vi "Initialize Attributes.vi"(8 "error in (no error)":errorcluster, 10 "Attribute Data":variant, 11 "CS++PVProxy in":refnum<class "CS++PVProxy.lvclass">) -> (0 "error out":errorcluster, 2 "Found?":bool, 3 "CS++PVProxy out":refnum<class "CS++PVProxy.lvclass">)   [LabVIEW 2015, in "CS++PVProxy.lvlib" / "CS++PVProxy.lvclass"]
doc: "Initialize object attribute.\n\nUnique resources should be allocated elsewhere!"
uses:
  CS++PVProxy.lvclass
  Classes/CS++ProcessVariables/ProcessVariable/PV.lvclass
  CS++PVMonitor Messages/CS++PVUpdate Msg/CS++PVUpdate Msg.lvclass
  CS++BaseActor/CS++BaseActor.lvclass/CS++BaseActor.ctl
  Classes/CS++ProcessVariables/ProcessVariable/PV.lvclass/PV.ctl
  Classes/CS++ProcessVariables/PVConnection/PVConnection.lvclass
  CS++PVMonitor Messages/CS++PVUpdate Msg/CS++PVUpdate Msg.lvclass/CS++PVUpdate Msg.ctl
  CS++PVProxy.lvclass/CS++PVProxy.ctl
  Classes/CS++ProcessVariables/ProcessVariable/Write Name.vi
  Classes/CS++ProcessVariables/ProcessVariable/Write PV URL.vi
  Classes/CS++ProcessVariables/ProcessVariable/Write Type Descriptor.vi
  <vilib>/Utility/error.llb/Error Cluster From Error Code.vi
  CS++BaseActor/CS++BaseActor.lvclass
  Classes/CS++BaseClasses/Factory/CS++Factory.lvclass
  Libraries/Utilities/CS++Utilities.lvlib
  Classes/CS++ProcessVariables/CS++ProcessVariables.lvlib
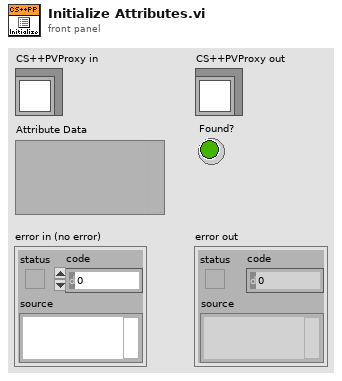
[diagram p1: front panel]
types:
  T1 = cluster{string, string, "CS++PVUpdate Msg out":refnum<class "CS++PVUpdate Msg.lvclass">, "CS++ProcessVariables.lvlib:PVConnection.lvclass":refnum<class "PVConnection.lvclass">}
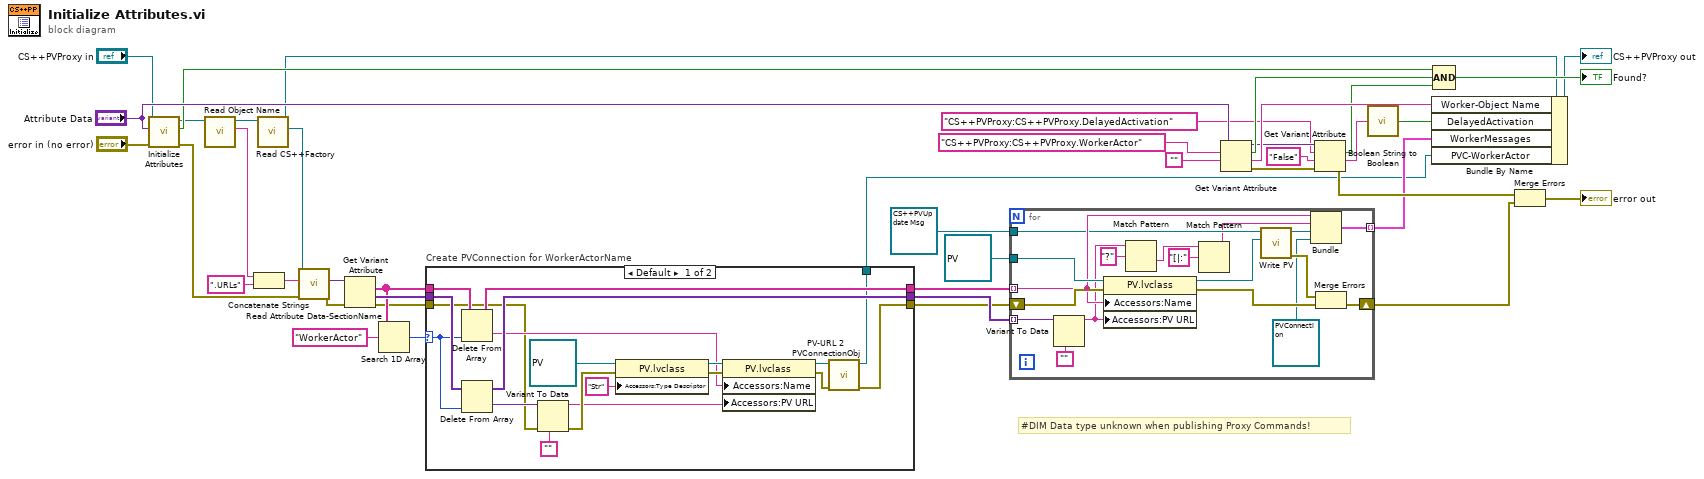
[diagram p0: block diagram]
diagram:
  # "#DIM Data type unknown when publishing Proxy Commands!"
  n1 = call-parent "Initialize Attributes.vi"("error in (no error)"="error in (no error)", "Attribute Data"="Attribute Data", "CS++BaseActor in"="CS++PVProxy in") -> ("error out"=w26:errorcluster, "Found?"=w34:bool, "CS++BaseActor out"=w31:refnum<class "CS++PVProxy.lvclass">)  [unwired: 6 in]
  n2 = call "Read Object Name.vi"("CS++BaseActor in"=w31) -> ("Object Name"=w27:string, "CS++BaseActor out"=w32:refnum<class "CS++PVProxy.lvclass">)  [unwired: 8 in, 1 out]
  n3 = Concatenate Strings(w27, ".URLs" ("string")) -> (w29:string)
  n4 = call "Read CS++Factory.vi"("CS++BaseActor in"=w32) -> ("CS++Factory"=w28:refnum<class "CS++Factory.lvclass">, "CS++BaseActor out"=w20:refnum<class "CS++PVProxy.lvclass">)  [unwired: 8 in, 1 out]
  n5 = call-dynamic "Read Attribute Data-SectionName.vi"("error in (no error)"=w26, "Object Name"=w29, "CS++Factory in"=w28) -> ("error out"=w24:errorcluster, "Attribute Data"=w23:variant)  [unwired: 6 in, 1 out]
  n6 = Get Variant Attribute(Variant=w23, error in=w24) -> (names=w7:string[], values=w9:variant[], error out=w3:errorcluster)  [unwired: 2 in, 1 out]
  n7 = Search 1D Array(1D array=w7, element="WorkerActor") -> (index of element=w5:i32)  [unwired: 1 in]
  n8 = case "Create PVConnection for WorkerActorName" shown="Default" w5 {
    selector: w5 -> [w57 _]
    tunnel: w9 -> [w61 w63]
    tunnel: [w60 w63] -> w8
    tunnel: w7 -> [w59 w64]
    tunnel: [w58 w64] -> w6
    tunnel: w3 -> [w47 w62]
    tunnel: [w45 w62] -> w2
    tunnel: [w44 _] -> w1
    frame Default {
      n9 = Delete From Array(array=w59, index=w57) -> (deleted portion=w48:string, array with subset deleted=w58:string[])  [unwired: 1 in]
      n10 = Delete From Array(array=w61, index=w57) -> (deleted portion=w49:variant, array with subset deleted=w60:variant[])  [unwired: 1 in]
      n11 = Variant To Data(error in=w47, type="", Variant=w49) -> (data=w43:string, error out=w46:errorcluster)
      n12 = property class="PV.lvclass"(reference=refnum<class "PV.lvclass"> refnum ("CS++ProcessVariables.lvlib:PV.lvclass"), error in=w46, "Accessors:Type Descriptor"="Str" ("Type Descriptor")) -> (reference out=w55:refnum<class "PV.lvclass">, error out=w56:errorcluster)
      n13 = property class="PV.lvclass"(reference=w55, error in=w56, "Accessors:Name"=w48, "Accessors:PV URL"=w43) -> (reference out=w53:refnum<class "PV.lvclass">, error out=w54:errorcluster)
      n14 = call "PV-URL 2 PVConnectionObj.vi"("Error In"=w54, "PV"=w53) -> ("Error Out"=w45:errorcluster, "PVConnection"=w44:refnum<class "PVConnection.lvclass">)  [unwired: 7 in, 1 out]
    }
    frame -1 {
    }
  }
  n15 = for {
    tunnel: refnum<class "PV.lvclass"> refnum ("CS++ProcessVariables.lvlib:PV.lvclass") -> [w82]
    shift-right: [w72] -> w22
    shift-left: w2 -> [w79]
    tunnel: w6 -> [w78] mode=indexing
    tunnel: w8 -> [w80] mode=indexing
    tunnel: [w77] -> w11 mode=indexing
    tunnel: refnum<class "CS++PVUpdate Msg.lvclass"> refnum ("CS++PVMonitor.lvlib:CS++PVUpdate Msg.lvclass") -> [w76]
    n16 = Variant To Data(type="", Variant=w80) -> (data=w68:string)  [unwired: 1 in, 1 out]
    n17 = property class="PV.lvclass"(reference=w82, error in=w79, "Accessors:Name"=w78, "Accessors:PV URL"=w68) -> (reference out=w74:refnum<class "PV.lvclass">, error out=w71:errorcluster)
    n18 = Match Pattern(string=w68, regular expression="?") -> (after substring=w65:string)  [unwired: 1 in, 3 out]
    n19 = Match Pattern(string=w65, regular expression="[|:") -> (before substring=w67:string)  [unwired: 1 in, 3 out]
    n20 = call "Write PV.vi"("PV"=w74, "CS++PVUpdate Msg in"=w76) -> ("error out"=w73:errorcluster, "CS++PVUpdate Msg out"=w75:refnum<class "CS++PVUpdate Msg.lvclass">)  [unwired: 8 in]
    n21 = Bundle(w78, w67, "CS++PVUpdate Msg out"=w75, "CS++ProcessVariables.lvlib:PVConnection.lvclass"=refnum<class "PVConnection.lvclass"> refnum) -> (w77:T1)  [unwired: 1 in]
    n22 = Merge Errors(w73, w71) -> (w72:errorcluster)
  }
  n23 = Get Variant Attribute(Variant="Attribute Data", name="CS++PVProxy:CS++PVProxy.WorkerActor", default value (empty Variant)="") -> (duplicate Variant=w16:variant, found=w33:bool, value=w35:string, error out=w18:errorcluster)  [unwired: 1 in]
  n24 = Get Variant Attribute(Variant=w16, name="CS++PVProxy:CS++PVProxy.DelayedActivation", default value (empty Variant)="False", error in=w18) -> (found=w12:bool, value=w13:string, error out=w17:errorcluster)  [unwired: 1 out]
  n25 = call "Boolean String to Boolean.vi"("T/F String"=w13) -> ("Value"=w10:bool)
  n26 = Bundle By Name(cluster=w20, "Worker-Object Name"=w35, "DelayedActivation"=w10, "WorkerMessages"=w11, "PVC-WorkerActor"=w1) -> (→"CS++PVProxy out":refnum<class "CS++PVProxy.lvclass">)
  n27 = Compound Arithmetic op=AND(w34, w33, w12) -> (→"Found?":bool)
  n28 = Merge Errors(w17, w22) -> (→"error out":errorcluster)
